vi "Build Rule.vi"(11 "String":string) -> (3 "Cluster":T1)   [LabVIEW 2023]
uses:
  Cluster_Rule.ctl
  ENUM_Compare.ctl
  ENUM_Value Type.ctl
  <vilib>/Utility/error.llb/Trim Whitespace One-Sided.vi
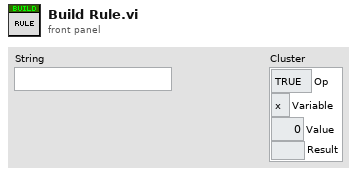
[diagram p1: front panel]
types:
  T1 = typedef "Cluster_Rule.ctl" = cluster{"Op":T2, "Variable":T3, "Value":i32, "Result":string}
  T2 = typedef "ENUM_Compare.ctl" = enum16{"TRUE", "<", ">", "<=", ">="}
  T3 = typedef "ENUM_Value Type.ctl" = enum16{"x", "m", "a", "s"}
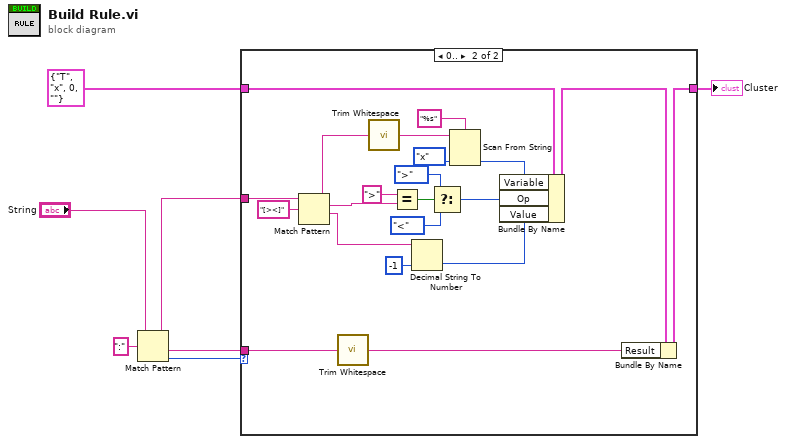
[diagram p0: block diagram]
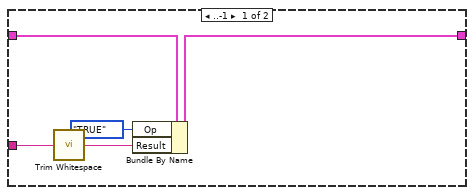
[diagram p2: hidden frame]
diagram:
  n1 = Match Pattern(string="String", regular expression=":") -> (before substring=w3:string, after substring=w4:string, offset past match=w1:i32)  [unwired: 1 in, 1 out]
  n2 = case shown="0.." w1 {
    tunnel: [w12 w33] -> w5
    tunnel: w4 -> [_ w32]
    tunnel: w3 -> [w10 w30]
    tunnel: T1 {"Op"=enum."TRUE", "Variable"=enum."x", "Value"=0, "Result"=""} ("Cluster") -> [w11 w26]
    frame ..-1 {
      n3 = call <vilib>:"Trim Whitespace.vi"("string"=w10) -> ("trimmed string"=w8:string)  [unwired: 1 in]
      n4 = Bundle By Name(cluster=w11, "Op"=ENUM_Compare."TRUE", "Result"=w8) -> (w12:T1)
    }
    frame 0.. {
      n5 = Match Pattern(string=w30, regular expression="[><]") -> (before substring=w28:string, match substring=w29:string, after substring=w27:string)  [unwired: 1 in, 1 out]
      n6 = call <vilib>:"Trim Whitespace.vi"("string"=w32) -> ("trimmed string"=w13:string)  [unwired: 1 in]
      n7 = call <vilib>:"Trim Whitespace.vi"("string"=w28) -> ("trimmed string"=w15:string)  [unwired: 1 in]
      n8 = Equal?(x=">", y=w29) -> (x = y?=w24:bool)
      n9 = Decimal String To Number(string=w27, default (0L)=-1 ("default (0 I32)")) -> (number=w19:i32)  [unwired: 1 in, 1 out]
      n10 = Select(t=ENUM_Compare.">" ("Compare"), s=w24, f=ENUM_Compare."<" ("Compare")) -> (s? t:f=w21:T2)
      n11 = Scan From String(format string="%s", input string=w15, default 1=ENUM_Value_Type."x" ("Value Type")) -> (output 1=w16:T3)  [unwired: 2 in, 3 out]
      n12 = Bundle By Name(cluster=w26, "Variable"=w16, "Op"=w21, "Value"=w19) -> (w25:T1)
      n13 = Bundle By Name(cluster=w25, "Result"=w13) -> (w33:T1)
    }
  }
  "Cluster" <- w5
